vi "[PointerArray] - Get Pointer.vi"(6 "Create If Not Found":bool=TRUE, 8 "Error":errorcluster, 9 "Pointer":refnum<class "_Pointer.lvclass">, 10 "Index":i32=-1, 11 "WavBuf":refnum<class "WavBuf.lvclass">) -> (0 "Error Out":errorcluster, 1 "Pointer Out":refnum<class "_Pointer.lvclass">, 2 "Index Out":i32, 3 "WavBuf Out":refnum<class "WavBuf.lvclass">, 4 "Found Out":bool)   [LabVIEW 2024, in "WavBuf.lvclass"]
uses:
  WavBuf.lvclass
  Pointer/_Pointer.lvclass
  WavBuf.lvclass/WavBuf.ctl
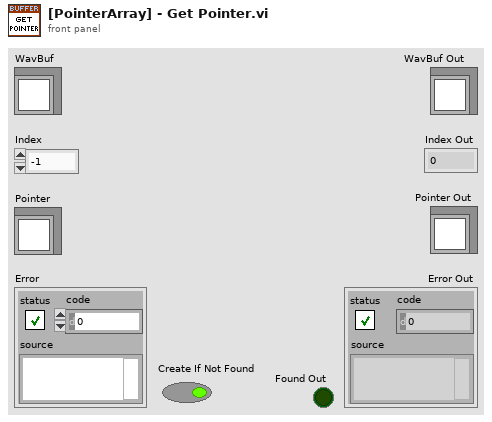
[diagram p1: front panel]
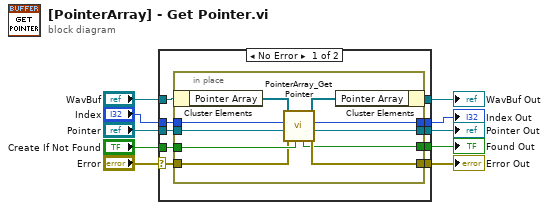
[diagram p0: block diagram]
diagram:
  n1 = case shown="No Error" "Error" {
    selector: "Error" -> [w13 w32]
    tunnel: [w12 w32] -> w9
    tunnel: [w19 w31] -> w7
    tunnel: "WavBuf" -> [w20 w31]
    tunnel: "Pointer" -> [w18 _]
    tunnel: "Index" -> [w17 _]
    tunnel: "Create If Not Found" -> [w16 _]
    tunnel: [w15 _] -> w3
    tunnel: [w14 _] -> w2
    tunnel: [w11 _] -> w1
    frame No Error {
      n2 = in-place {
        in-place-border: w18 -> [w29]
        in-place-border: w17 -> [w28]
        in-place-border: w16 -> [w27]
        in-place-border: [w25] -> w15
        in-place-border: [w24] -> w14
        in-place-border: w13 -> [w23]
        in-place-border: [w22] -> w12
        in-place-border: [w21] -> w11
        n3 = in-place-cluster #1(w20) -> ("Pointer Array"=w30:refnum<class "_Pointer.lvclass">[])
        n4 = call "PointerArray_Get Pointer.vi"("Create If Not Found"=w27, "Error"=w23, "Pointer"=w29, "Index"=w28, "Pointer Array"=w30) -> ("Error Out"=w22:errorcluster, "Pointer Out"=w25:refnum<class "_Pointer.lvclass">, "Index Out"=w24:i32, "Pointer Array Out"=w26:refnum<class "_Pointer.lvclass">[], "Found Out"=w21:bool)  [unwired: 2 in]
        n5 = in-place-cluster #1("Pointer Array"=w26) -> (w19:refnum<class "WavBuf.lvclass">)
      }
    }
    frame Error {
    }
  }
  "Error Out" <- w9
  "WavBuf Out" <- w7
  "Pointer Out" <- w3
  "Index Out" <- w2
  "Found Out" <- w1
